vi "makeDecisions.vi"(8 "error in (no error)":errorcluster, 10 "model":refnum<class "Model.lvclass">, 11 "MovingToNewForceState in":refnum<class "MovingToNewForceState.lvclass">) -> (0 "error out":errorcluster, 2 "model 2":refnum<class "Model.lvclass">, 3 "MovingToNewForceState out":refnum<class "MovingToNewForceState.lvclass">)   [LabVIEW 2015, in "MovingToNewForceState.lvclass"]
uses:
  MovingToNewForceState.lvclass
  Model/Model/Model.lvclass
  Typedefs/StateSelector.ctl
  Typedefs/M1M3SSSTypedefs.lvlib
  ExecutingCycleState/ExecutingCycleState.lvclass
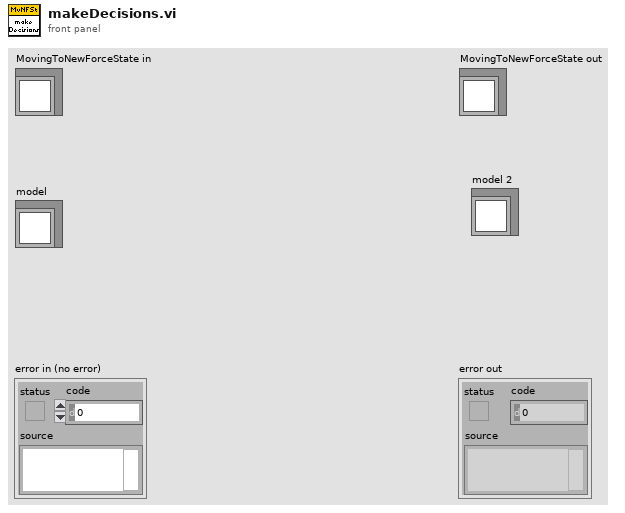
[diagram p1: front panel]
types:
  T1 = typedef "M1M3SSSTypedefs.lvlib/StateSelector.ctl" = enum16{"FaultState", "OffState", "RampingUpPressurePState", "RampingUpPressureSTState", "StandbyState", "StoppedState", "WaitingForSettledPState", "WaitingForSettledSTState"}
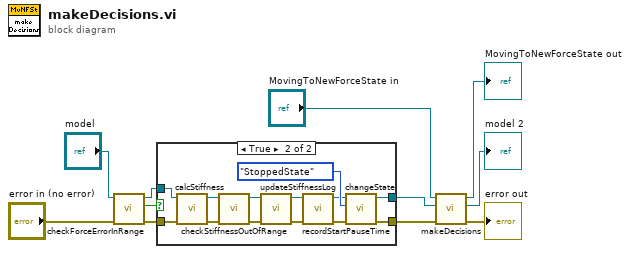
[diagram p0: block diagram]
diagram:
  n1 = call "checkForceErrorInRange.vi"("error in (no error)"="error in (no error)", "Model in"="model") -> ("error out"=w3:errorcluster, "inRangeIsTrue"=w4:bool, "Model out"=w5:refnum<class "Model.lvclass">)  [unwired: 7 in]
  n2 = case shown="True" w4 {
    tunnel: w5 -> [w13 w21]
    tunnel: w3 -> [w12 w20]
    tunnel: [w12 w26] -> w2
    tunnel: [w13 w25] -> w1
    frame False {
    }
    frame True {
      n3 = call "calcStiffness.vi"("error in (no error)"=w20, "Model in"=w21) -> ("error out"=w16:errorcluster, "Model out"=w17:refnum<class "Model.lvclass">)  [unwired: 8 in]
      n4 = call "checkStiffnessOutOfRange.vi"("error in (no error)"=w16, "Model in"=w17) -> ("error out"=w14:errorcluster, "Model out"=w15:refnum<class "Model.lvclass">)  [unwired: 7 in, 1 out]
      n5 = call "updateStiffnessLog.vi"("error in (no error)"=w14, "Model in"=w15) -> ("error out"=w18:errorcluster, "Model out"=w19:refnum<class "Model.lvclass">)  [unwired: 8 in]
      n6 = call "recordStartPauseTime.vi"("error in (no error)"=w18, "Model in"=w19) -> ("error out"=w22:errorcluster, "Model out"=w23:refnum<class "Model.lvclass">)  [unwired: 8 in]
      n7 = call "changeState.vi"("error in (no error)"=w22, "State:"=StateSelector."StoppedState", "Model in"=w23) -> ("error out"=w26:errorcluster, "Model out"=w25:refnum<class "Model.lvclass">)  [unwired: 7 in]
    }
  }
  n8 = call-parent "makeDecisions.vi"("error in (no error)"=w2, "model"=w1, "EnabledState in"="MovingToNewForceState in") -> ("error out"=→"error out":errorcluster, "model 2"=→"model 2":refnum<class "Model.lvclass">, "EnabledState out"=→"MovingToNewForceState out":refnum<class "MovingToNewForceState.lvclass">)  [unwired: 6 in]
